vi "DSF.Engine.Framework.Initialize.Transfer Groups.Split Rx and Tx.vi"(8 "error in (no error)":errorcluster, 11 "Framework in":refnum<class "Framework.lvclass">) -> (0 "error out":errorcluster, 3 "Framework out":refnum<class "Framework.lvclass">)   [LabVIEW 2017, in "DSF.Engine.lvlib" / "Framework.lvclass"]
uses:
  Framework.lvclass
  Transfer/DSF.Engine.Transfer Group.lvclass
  Framework.lvclass/Framework.ctl
  Transfer/DSF.Engine.Transfer Group.lvclass/DSF.Engine.Transfer Group.ctl
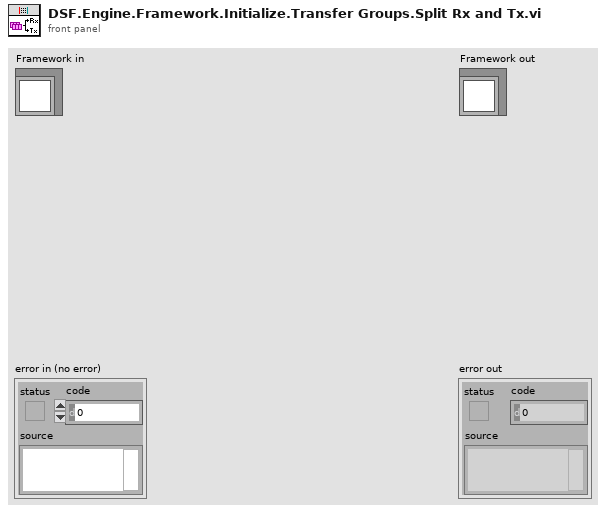
[diagram p1: front panel]
types:
  T1 = typedef "DSF.Shared.lvlib/DSF.Shared.Typedefs.Direction.ctl" = enum8{"Tx", "Rx"}
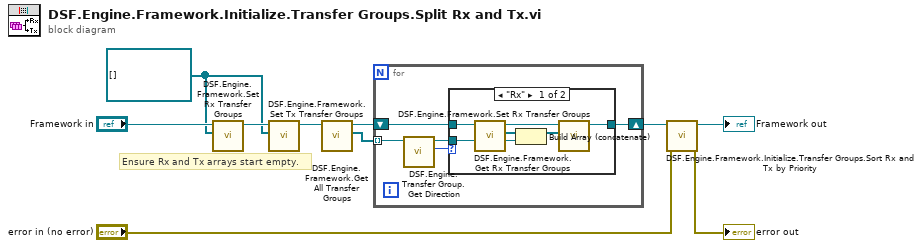
[diagram p0: block diagram]
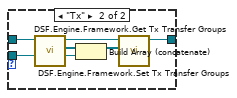
[diagram p2: hidden frame]
diagram:
  w8 = refnum<class "DSF.Engine.Transfer Group.lvclass">[] [] ("Rx Transfer Groups")
  # "Ensure Rx and Tx arrays start empty."
  n1 = call "DSF.Engine.Framework.Set Rx Transfer Groups.vi"("Rx Transfer Groups"=w8, "Framework in"="Framework in") -> ("Framework out"=w9:refnum<class "Framework.lvclass">)  [unwired: 9 in]
  n2 = call "DSF.Engine.Framework.Set Tx Transfer Groups.vi"("Tx Transfer Groups"=w8, "Framework in"=w9) -> ("Framework out"=w7:refnum<class "Framework.lvclass">)  [unwired: 9 in]
  n3 = call "DSF.Engine.Framework.Get All Transfer Groups.vi"("Framework in"=w7) -> ("All Transfer Groups"=w5:refnum<class "DSF.Engine.Transfer Group.lvclass">[], "Framework out"=w6:refnum<class "Framework.lvclass">)  [unwired: 9 in]
  n4 = for {
    tunnel: w5 -> [w15] mode=indexing
    shift-right: [w11] -> w4
    shift-left: w6 -> [w13]
    n5 = call "DSF.Engine.Transfer Group.Get Direction.vi"("Transfer Group in"=w15) -> ("Direction"=w14:T1, "Transfer Group out"=w12:refnum<class "DSF.Engine.Transfer Group.lvclass">)  [unwired: 9 in]
    n6 = case shown="\"Rx\"" w14 {
      tunnel: w13 -> [w21 w26]
      tunnel: w12 -> [w19 w27]
      tunnel: [w16 w24] -> w11
      frame "Rx" {
        n7 = call "DSF.Engine.Framework.Get Rx Transfer Groups.vi"("Framework in"=w21) -> ("Rx Transfer Groups"=w20:refnum<class "DSF.Engine.Transfer Group.lvclass">[], "Framework out"=w18:refnum<class "Framework.lvclass">)  [unwired: 9 in]
        n8 = Build Array (concatenate)(w20, w19) -> (w17:refnum<class "DSF.Engine.Transfer Group.lvclass">[])
        n9 = call "DSF.Engine.Framework.Set Rx Transfer Groups.vi"("Rx Transfer Groups"=w17, "Framework in"=w18) -> ("Framework out"=w16:refnum<class "Framework.lvclass">)  [unwired: 9 in]
      }
      frame "Tx" {
        n10 = call "DSF.Engine.Framework.Get Tx Transfer Groups.vi"("Framework in"=w26) -> ("Tx Transfer Groups"=w22:refnum<class "DSF.Engine.Transfer Group.lvclass">[], "Framework out"=w25:refnum<class "Framework.lvclass">)  [unwired: 9 in]
        n11 = Build Array (concatenate)(w22, w27) -> (w23:refnum<class "DSF.Engine.Transfer Group.lvclass">[])
        n12 = call "DSF.Engine.Framework.Set Tx Transfer Groups.vi"("Tx Transfer Groups"=w23, "Framework in"=w25) -> ("Framework out"=w24:refnum<class "Framework.lvclass">)  [unwired: 9 in]
      }
    }
  }
  n13 = call "DSF.Engine.Framework.Initialize.Transfer Groups.Sort Rx and Tx by Priority.vi"("error in (no error)"="error in (no error)", "Framework in"=w4) -> ("error out"=→"error out":errorcluster, "Framework out"=→"Framework out":refnum<class "Framework.lvclass">)  [unwired: 8 in]
